vi "Write ClassName.vi"(8 "error in (no error)":errorcluster, 10 "ClassName":string, 11 "GObject in":refnum<class "GObject.lvclass">) -> (0 "error out":errorcluster, 3 "GObject out":refnum<class "GObject.lvclass">)   [LabVIEW 2013, in "SET Project Data.lvlib" / "GObject.lvclass"]
uses:
  GObject.lvclass
  GObject.lvclass/GObject.ctl
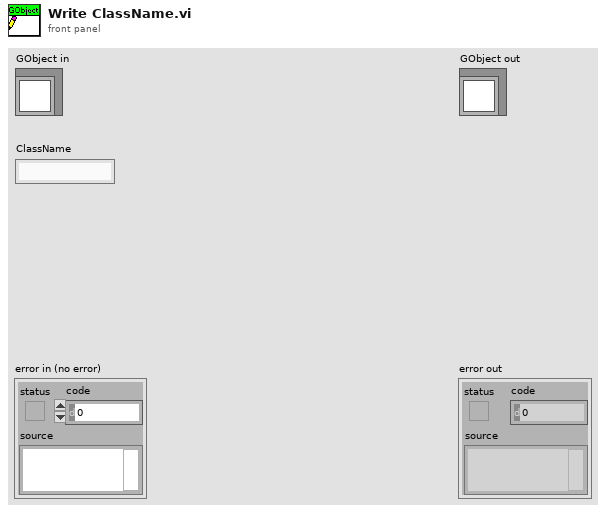
[diagram p1: front panel]
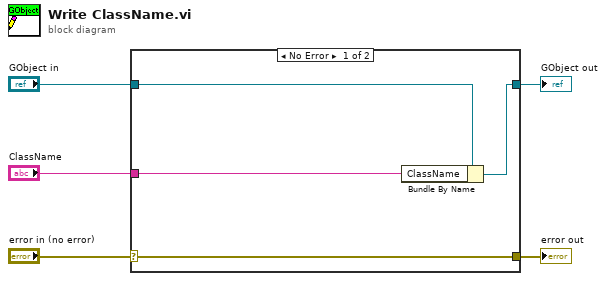
[diagram p0: block diagram]
diagram:
  n1 = case shown="No Error" "error in (no error)" {
    selector: "error in (no error)" -> [w9 w10]
    tunnel: [w9 w10] -> w4
    tunnel: [w7 w11] -> w2
    tunnel: "GObject in" -> [w8 w11]
    tunnel: "ClassName" -> [w6 _]
    frame No Error {
      n2 = Bundle By Name(cluster=w8, "ClassName"=w6) -> (w7:refnum<class "GObject.lvclass">)
    }
    frame Error {
    }
  }
  "error out" <- w4
  "GObject out" <- w2
